vi "HandleScore.vi"(8 "error in (no error)":errorcluster, 10 "Engine in":refnum<class "Engine.lvclass">, 11 "Bouncer in":refnum<class "Bouncer.lvclass">) -> (0 "error out":errorcluster, 2 "Engine out":refnum<class "Engine.lvclass">, 3 "Bouncer out":refnum<class "Bouncer.lvclass">)   [LabVIEW 2019, in "RT_Game.lvlib" / "Bouncer.lvclass"]
uses:
  Bouncer.lvclass
  C:/Users/FreshBob/Dropbox/VIs/myRIO_GameConsole/RT/RT_Game/Game/Game.lvclass
  Engine/Engine.lvclass
  Game/Game.lvclass/Game.ctl
  Bouncer.lvclass/Bouncer.ctl
  Menu/States.ctl
  BounceTarget/BounceTarget.lvclass/BounceTarget.ctl
  GameObject/GameObject.lvclass/GameObject.ctl
  Game/Write State.vi
  BounceTarget/Write Lives.vi
  GameObject/Write IsActive.vi
  BounceTarget/Write DoDraw.vi
  Game/Read Player1Score.vi
  Game/Read Player2Score.vi
  Game/Write Player1Score.vi
  Game/Write Player2Score.vi
  BounceTarget/BounceTarget.lvclass
  C:/Users/FreshBob/Dropbox/VIs/myRIO_GameConsole/RT/RT_Game/GameObject/GameObject.lvclass
  PongBall/PongBall.lvclass
  Game/Game.lvclass
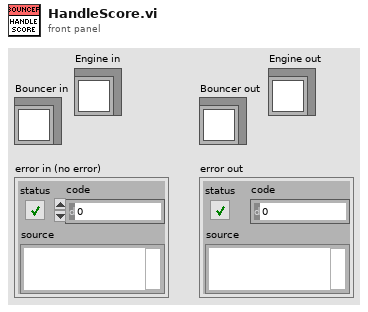
[diagram p1: front panel]
types:
  T1 = enum16{"all", "up", "down", "left", "right", "leftup", "rightup", "leftdown", "rightdown"}
  T2 = typedef "RT_Game.lvlib/Game.lvclass/States.ctl" = enum16{"Init", "Restart", "Menu", "Game", "Resume", "ToggleSingleplayer", "LoadNextGame", "ExitToMenu", "NewHighscore", "GameOver", "SlideOut"}
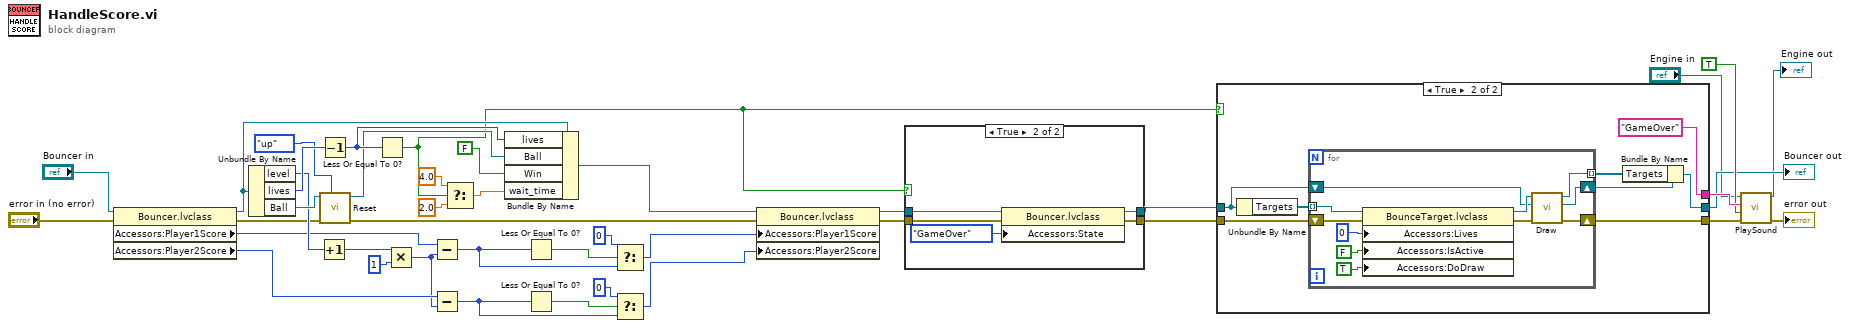
[diagram p0: block diagram]
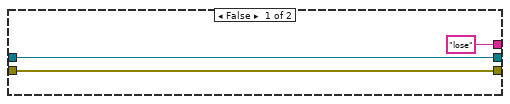
[diagram p3: hidden frame]
diagram:
  n1 = property class="Bouncer.lvclass"(reference="Bouncer in", error in="error in (no error)") -> (reference out=w15:refnum<class "Bouncer.lvclass">, error out=w17:errorcluster, "Accessors:Player1Score"=w14:i32, "Accessors:Player2Score"=w11:i32)
  n2 = Unbundle By Name(w15) -> ("level"=w22:i16, "lives"=w36:i16, "Ball"=w34:refnum<class "PongBall.lvclass">)
  n3 = Increment(x=w22) -> (x+1=w21:i16)
  n4 = Decrement(x=w36) -> (x-1=w37:i16)
  n5 = call "Reset.vi"("Direction (all)"=T1."up", "error in (no error)"=w17, "PongBall in"=w34) -> ("error out"=w33:errorcluster, "PongBall out"=w35:refnum<class "PongBall.lvclass">)  [unwired: 7 in]
  n6 = Less Or Equal To 0?(x=w37) -> (x <= 0?=w4:bool)
  n7 = Multiply(x=w21, y=i16 1 ("x")) -> (x*y=w10:i16)
  n8 = Subtract(x=w14, y=w10) -> (x-y=w28:i32)
  n9 = Subtract(x=w11, y=w10) -> (x-y=w12:i32)
  n10 = Select(t=4.0, s=w4, f=2.0 ("wait_time")) -> (s? t:f=w40:dbl)
  n11 = Bundle By Name(cluster=w15, "lives"=w37, "Ball"=w35, "Win"=FALSE, "wait_time"=w40) -> (w19:refnum<class "Bouncer.lvclass">)
  n12 = Less Or Equal To 0?(x=w28) -> (x <= 0?=w27:bool)
  n13 = Less Or Equal To 0?(x=w12) -> (x <= 0?=w13:bool)
  n14 = Select(t=i16 0, s=w27, f=w28) -> (s? t:f=w18:i32)
  n15 = Select(t=i16 0, s=w13, f=w12) -> (s? t:f=w9:i32)
  n16 = property class="Bouncer.lvclass"(reference=w19, error in=w33, "Accessors:Player1Score"=w18, "Accessors:Player2Score"=w9) -> (reference out=w6:refnum<class "Bouncer.lvclass">, error out=w20:errorcluster)
  n17 = case shown="True" w4 {
    tunnel: w20 -> [w42 w48]
    tunnel: [w42 w47] -> w7
    tunnel: w6 -> [w43 w46]
    tunnel: [w43 w45] -> w5
    frame False {
    }
    frame True {
      n18 = property class="Bouncer.lvclass"(reference=w46, error in=w48, "Accessors:State"=States."GameOver" ("State")) -> (reference out=w45:refnum<class "Bouncer.lvclass">, error out=w47:errorcluster)
    }
  }
  n19 = case shown="True" w4 {
    tunnel: w7 -> [w50 w56]
    tunnel: [w50 w55] -> w30
    tunnel: w5 -> [w51 w57]
    tunnel: [w51 w54] -> w3
    tunnel: ["lose" ("Name") "GameOver" ("Name")] -> w25
    frame False {
    }
    frame True {
      n20 = Unbundle By Name(w57) -> ("Targets"=w59:refnum<class "BounceTarget.lvclass">[])
      n21 = for {
        tunnel: w59 -> [w68] mode=indexing
        tunnel: [w64] -> w58 mode=indexing
        shift-right: [w66] -> w55
        shift-left: w56 -> [w70]
        shift-right: [w63] -> w52
        shift-left: w57 -> [w60]
        n22 = property class="BounceTarget.lvclass"(reference=w68, error in=w70, "Accessors:Lives"=i16 0 ("Lives"), "Accessors:IsActive"=FALSE ("IsActive"), "Accessors:DoDraw"=TRUE ("DoDraw")) -> (reference out=w65:refnum<class "BounceTarget.lvclass">, error out=w69:errorcluster)
        n23 = call "Draw.vi"("error in (no error)"=w69, "RT_Game.lvlib:Game.lvclass"=w60, "BounceTarget in"=w65) -> ("error out"=w66:errorcluster, "RT_Game.lvlib:Game.lvclass 2"=w63:refnum<class "Bouncer.lvclass">, "BounceTarget out"=w64:refnum<class "BounceTarget.lvclass">)  [unwired: 6 in]
      }
      n24 = Bundle By Name(cluster=w52, "Targets"=w58) -> (w54:refnum<class "Bouncer.lvclass">)
    }
  }
  "Bouncer out" <- w3
  n25 = call "PlaySound.vi"("error in (no error)"=w30, "Overwrite"=TRUE, "Name"=w25, "Engine in"="Engine in") -> ("error out"=→"error out":errorcluster, "Engine out"=→"Engine out":refnum<class "Engine.lvclass">)  [unwired: 6 in]
